vi "Teleop.vi"(10 "Match Info":T1={"Autonomous Elapsed Seconds"=0.0, "TeleOp Elapsed Seconds"=0.0, "Disabled Elapsed Seconds"=0.0, "Visited Autonomous"=FALSE, "Visited TeleOp"=FALSE, "Visited Disabled"=FALSE, "Autonomous Settings"={"Autonomous Style"=enum."Independent", "VI Refnum"=refnum}}, 11 "Call Context":T2) -> ()   [LabVIEW 2017]
doc: "This VI is called for each TeleOp packet received from the DS where the robot is not disabled. It is often used to read from the joysticks and update I/O or to update setpoints for timed control loops. It should complete and return within 20 milliseconds or it may miss DS packets."
uses:
  <vilib>/Rock Robotics/WPI/DriverStation/WPI_DriverStationDerivedRobotMode.ctl
  <vilib>/Rock Robotics/WPI/DriverStation/WPI_DriverStationMatch Info.ctl
  <vilib>/Rock Robotics/WPI/Solenoid/WPI_SolenoidValue.ctl
  <vilib>/Rock Robotics/WPI/Utilities/WPI_GetSetVariantRefNum.vi
  Robot Global Data.vi
  <vilib>/Rock Robotics/Network Tables/NT Read Boolean.vi
  <vilib>/Rock Robotics/Network Tables/NT Read Number.vi
  <vilib>/Rock Robotics/WPI/Solenoid/WPI_SolenoidSetEnum.vi
  <vilib>/Rock Robotics/Network Tables/NT Write Numeric Array.vi
  <vilib>/Rock Robotics/Network Tables/NT Write Boolean Array.vi
panel:
  out "Sample Slider 0":dbl(slide) scale=0.0..5.0
  out "Sample Boolean 1":bool
  out "Sample Boolean 0":bool
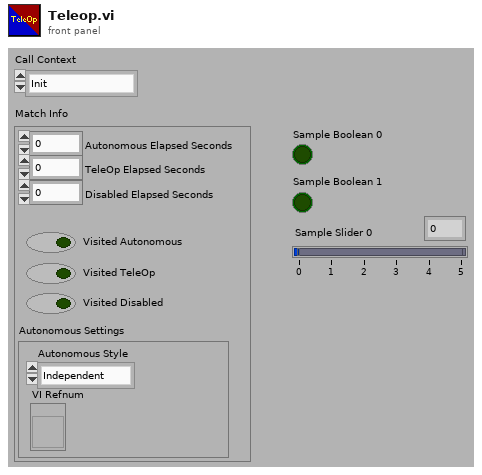
[diagram p1: front panel]
types:
  T1 = typedef "WPI_DriverStationMatch Info.ctl" = cluster{"Autonomous Elapsed Seconds":dbl, "TeleOp Elapsed Seconds":dbl, "Disabled Elapsed Seconds":dbl, "Visited Autonomous":bool, "Visited TeleOp":bool, "Visited Disabled":bool, "Autonomous Settings":cluster{"Autonomous Style":enum16{"Iterative", "Independent"}, "VI Refnum":refnum<vi>}}
  T2 = typedef "WPI_DriverStationDerivedRobotMode.ctl" = enum16{"Init", "Execute", "Stop"}
  T3 = typedef "WPI_SolenoidValue.ctl" = enum16{"Off", "On", "Forward", "Reverse"}
  T4 = typedef "WPI_SolenoidDevRef.ctl" = cluster{"DevStatus":errorcluster, "Pneumatics Control Module":u8, "Forward Solenoid Channel":T5, "Reverse Solenoid Channel":T5}
  T5 = typedef "WPI_SolenoidChannel.ctl" = enum8{"Solenoid 0", "Solenoid 1", "Solenoid 2", "Solenoid 3", "Solenoid 4", "Solenoid 5", "Solenoid 6", "Solenoid 7", "Invalid"}
  T6 = typedef "WPI_JoystickDevRef.ctl" = cluster{"Device":T7}
  T7 = typedef "WPI_JoystickDeviceEnum.ctl" = enum16{"USB 0", "USB 1", "USB 2", "USB 3", "USB 4", "USB 5"}
  T8 = typedef "WPI_RobotDriveDevRef.ctl" = cluster{"DevStatus":errorcluster, "Motors[]":T9[], "Square Inputs":bool, "Max Output":dbl}
  T9 = typedef "WPI_MotorControlDeviceRef.ctl" = cluster{"DeviceStatus":errorcluster, "Type":T10, "PWM":cluster{"PWM Channel":T11, "DeadBand":T12}, "CAN":cluster{"Device Number":u8, "SetOutput VI Ref":variant, "GetOutput VI Ref":variant, "Enable VI Ref":variant, "Disable VI Ref":variant, "Data":variant}, "Invert":bool, "DIO PWM":cluster{"PWM \"Enable\" Channel":T11, "DIOChannel":T13, "PWM Rate":dbl}}
  T10 = typedef "WPI_MotorControlType.ctl" = enum16{"PWM", "CAN", "DIO PWM"}
  T11 = typedef "FPGA_DIOPWMChannel.ctl" = enum8{"PWM 0", "PWM 1", "PWM 2", "PWM 3", "PWM 4", "PWM 5", "PWM 6", "PWM 7", "PWM 8", "PWM 9", "PWM MXP 0", "PWM MXP 1", "PWM MXP 2", "PWM MXP 3", "PWM MXP 4", "PWM MXP 5", "PWM MXP 6", "PWM MXP 7", "PWM MXP 8", "PWM MXP 9", "Invalid"}
  T12 = typedef "WPI_PWMDeadband.ctl" = cluster{"Name":string, "maxPositivePwm":i32, "minPositivePwm":i32, "centerPwm":i32, "maxNegativePwm":i32, "minNegativePwm":i32, "angularRange":u16}
  T13 = typedef "FPGA_DIOChannel.ctl" = enum8{"DIO 0", "DIO 1", "DIO 2", "DIO 3", "DIO 4", "DIO 5", "DIO 6", "DIO 7", "DIO 8", "DIO 9", "DIO MXP 0", "DIO MXP 1", "DIO MXP 2", "DIO MXP 3", "DIO MXP 4", "DIO MXP 5", "DIO MXP 6", "DIO MXP 7", "DIO MXP 8", "DIO MXP 9", "DIO MXP 10", "DIO MXP 11", "DIO MXP 12", "DIO MXP 13", "DIO MXP 14", "DIO MXP 15", "SPI Port CS1", "SPI Port CS2", "SPI Port CS3", "SPI Port MISO", "SPI Port MOSI", "Invalid"}
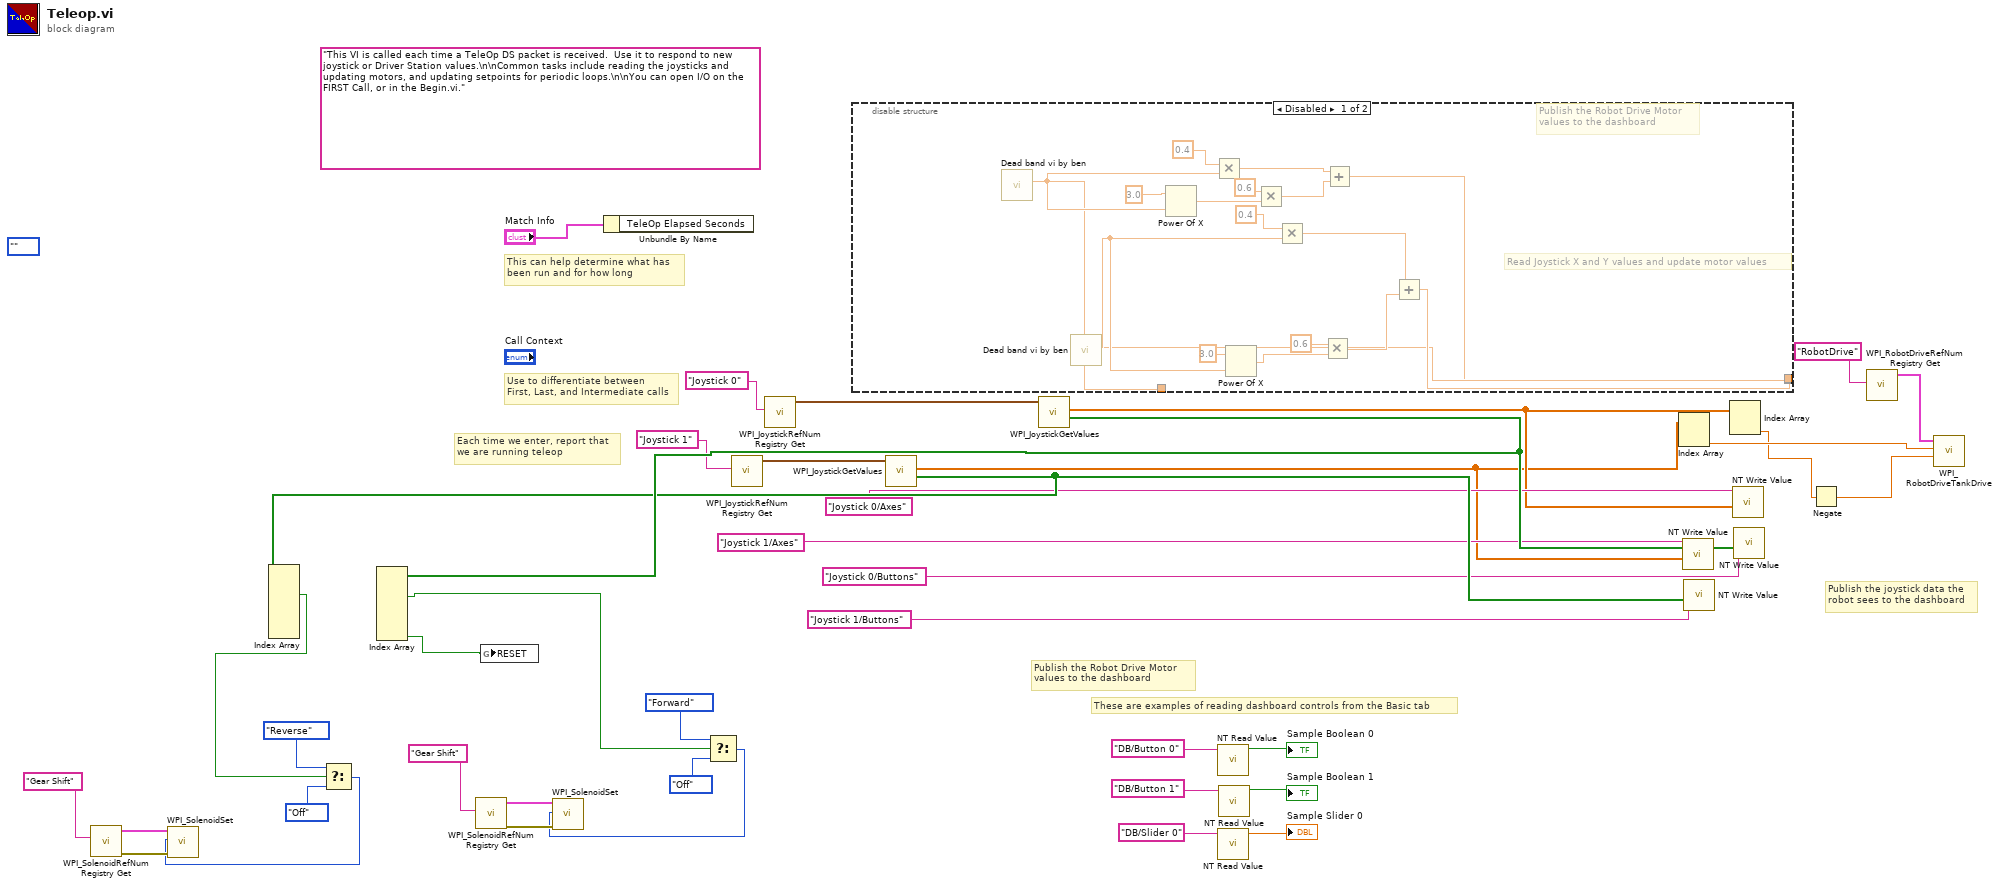
[diagram p0: block diagram]
diagram:
  (unwired) enum16{""}.""
  (unwired) "This VI is called each time a TeleOp DS packet is received.  Use it to respond to new joystick or Driver Station values.\n\nCommon tasks include reading the joysticks and updating motors, and updating setpoints for periodic loops.\n\nYou can open I/O on the FIRST Call, or in the Begin.vi."
  # "Publish the Robot Drive Motor\nvalues to the dashboard"
  # "Publish the joystick data the\nrobot sees to the dashboard"
  # "These are examples of reading dashboard controls from the Basic tab"
  # "Each time we enter, report that\nwe are running teleop"
  # "Use to differentiate between\nFirst, Last, and Intermediate calls"
  # "This can help determine what has\nbeen run and for how long"
  n1 = call <vilib>:"WPI_SolenoidRefNum Registry Get.vi"("refnum name"="Gear Shift") -> ("error out"=w20:errorcluster, "SolenoidDevRef"=w21:T4)  [unwired: 9 in]
  n2 = call <vilib>:"WPI_SolenoidRefNum Registry Get.vi"("refnum name"="Gear Shift") -> ("error out"=w29:errorcluster, "SolenoidDevRef"=w30:T4)  [unwired: 9 in]
  n3 = Unbundle By Name("Match Info") -> ()  [unwired: 1 out]
  n4 = call <vilib>:"WPI_JoystickRefNum Registry Get.vi"("refnum name"="Joystick 1") -> ("JoystickDevRef"=w9:T6)  [unwired: 1 in, 9 out]
  n5 = call <vilib>:"WPI_JoystickRefNum Registry Get.vi"("refnum name"="Joystick 0") -> ("JoystickDevRef"=w38:T6)  [unwired: 1 in, 9 out]
  n6 = disable-structure shown="Disabled" {
    disable-tunnel: [w51 _] -> _
    disable-tunnel: _ -> [w42 _]
    disable-tunnel: _ -> [w41 _]
    disable-tunnel: [w40 _] -> _
    frame Disabled {
      # "Read Joystick X and Y values and update motor values"
      # "Publish the Robot Drive Motor\nvalues to the dashboard"
      n7 = call "Dead band vi by ben.vi"("Numeric"=w41) -> ("Deadbanded Value"=w44:dbl)  [unwired: 10 in]
      n8 = call "Dead band vi by ben.vi"("Numeric"=w42) -> ("Deadbanded Value"=w53:dbl)  [unwired: 10 in]
      n9 = Power Of X(1:w44, 2:3.0 ("y")) -> (0:w49:dbl)
      n10 = Multiply(x=0.4, y=w44) -> (x*y=w47:dbl)
      n11 = Power Of X(1:w53, 2:3.0 ("y")) -> (0:w56:dbl)
      n12 = Multiply(x=0.6, y=w49) -> (x*y=w48:dbl)
      n13 = Multiply(x=0.4, y=w53) -> (x*y=w54:dbl)
      n14 = Multiply(x=0.6, y=w56) -> (x*y=w55:dbl)
      n15 = Add(x=w47, y=w48) -> (x+y=w40:dbl)
      n16 = Add(x=w54, y=w55) -> (x+y=w51:dbl)
    }
    frame Enabled {
    }
  }
  n17 = call <vilib>:"WPI_JoystickGetValues.vi"("JoystickDevRef"=w9) -> ("Buttons"=w22:bool[], "Axes"=w5:dbl[])  [unwired: 6 in, 3 out]
  n18 = Index Array(array=w22) -> (element #2=w16:bool)  [unwired: 7 in, 6 out]
  n19 = Select(t=WPI_SolenoidValue."Reverse" ("Value"), s=w16, f=WPI_SolenoidValue."Off" ("Value")) -> (s? t:f=w15:T3)
  n20 = call-poly <vilib>:"WPI_SolenoidSet.vi"("error in (no error)"=w20, "Value"=w15, "SolenoidDevRef"=w21) -> ()  [unwired: 7 in, 2 out]
  n21 = call <vilib>:"WPI_JoystickGetValues.vi"("JoystickDevRef"=w38) -> ("Buttons"=w24:bool[], "Axes"=w12:dbl[])  [unwired: 6 in, 3 out]
  n22 = Index Array(array=w24) -> (element #2=w23:bool, element #7=w4:bool)  [unwired: 7 in, 5 out]
  n23 = global write "Robot Global Data.vi" "RESET"(w4) -> ()
  n24 = Select(t=WPI_SolenoidValue."Forward" ("Value"), s=w23, f=WPI_SolenoidValue."Off" ("Value")) -> (s? t:f=w25:T3)
  n25 = call-poly <vilib>:"WPI_SolenoidSet.vi"("error in (no error)"=w29, "Value"=w25, "SolenoidDevRef"=w30) -> ()  [unwired: 7 in, 2 out]
  n26 = call-poly <vilib>:"NT Read Value.vi"("Name"="DB/Button 0" ("refnum name")) -> ("Boolean"=→"Sample Boolean 0":bool)  [unwired: 9 in, 1 out]
  n27 = call-poly <vilib>:"NT Read Value.vi"("Name"="DB/Slider 0" ("refnum name")) -> ("Numeric"=→"Sample Slider 0":dbl)  [unwired: 9 in, 1 out]
  n28 = call-poly <vilib>:"NT Read Value.vi"("Name"="DB/Button 1" ("refnum name")) -> ("Boolean"=→"Sample Boolean 1":bool)  [unwired: 9 in, 1 out]
  n29 = Index Array(array=w5) -> (element #2=w3:dbl)  [unwired: 2 in, 1 out]
  n30 = call-poly <vilib>:"NT Write Value.vi"("Numeric Array"=w5, "Name"="Joystick 1/Axes") -> ()  [unwired: 9 in, 1 out]
  n31 = call-poly <vilib>:"NT Write Value.vi"("Boolean Array"=w22, "Name"="Joystick 1/Buttons") -> ()  [unwired: 9 in, 1 out]
  n32 = Index Array(array=w12) -> (element #2=w2:dbl)  [unwired: 2 in, 1 out]
  n33 = call-poly <vilib>:"NT Write Value.vi"("Numeric Array"=w12, "Name"="Joystick 0/Axes") -> ()  [unwired: 9 in, 1 out]
  n34 = call-poly <vilib>:"NT Write Value.vi"("Boolean Array"=w24, "Name"="Joystick 0/Buttons") -> ()  [unwired: 9 in, 1 out]
  n35 = Negate(x=w2) -> (-x=w1:dbl)
  n36 = call <vilib>:"WPI_RobotDriveRefNum Registry Get.vi"("refnum name"="RobotDrive") -> ("RobotDriveDevRef"=w11:T8)  [unwired: 9 in, 1 out]
  n37 = call <vilib>:"WPI_RobotDriveTankDrive.vi"("Right axis value"=w1, "Left axis value"=w3, "RobotDriveDevRef"=w11) -> ()  [unwired: 6 in, 3 out]
